vi "linear_backward.vi"(4 "cache":T1, 5 "dZ":dbl[][](array[numeric])) -> (0 "db":dbl[][](array[numeric]), 1 "dW":dbl[][](array[numeric]), 2 "dA_prev":dbl[][](array[numeric]))   [LabVIEW 2020]
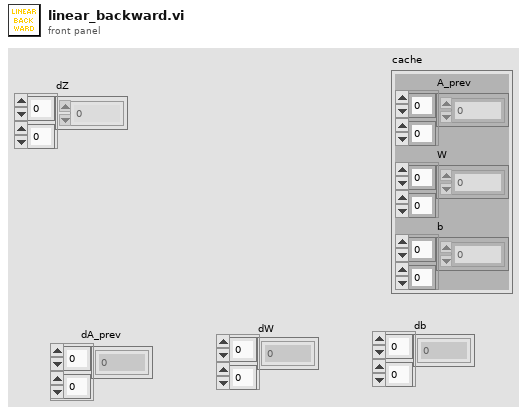
[diagram p1: front panel]
types:
  T1 = cluster{"A_prev":dbl[][], "W":dbl[][], "b":dbl[][]}
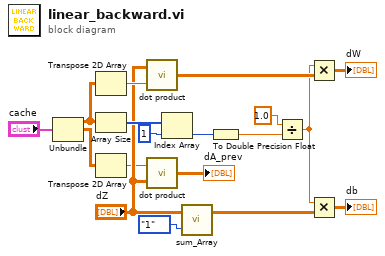
[diagram p0: block diagram]
diagram:
  n1 = Unbundle("cache") -> ("A_prev"=w12:dbl[][], "W"=w6:dbl[][])  [unwired: 1 out]
  n2 = Transpose 2D Array(2D array=w12) -> (transposed array=w11:dbl[][])
  n3 = Array Size(array=w12) -> (size(s)=w17:i32[])
  n4 = Transpose 2D Array(2D array=w6) -> (transposed array=w5:dbl[][])
  n5 = call "dot product.vi"("y"=w11, "x"="dZ") -> ("dot(x,y)"=w10:dbl[][])
  n6 = call "dot product.vi"("y"="dZ", "x"=w5) -> ("dot(x,y)"=→"dA_prev":dbl[][])
  n7 = Index Array(array=w17, index=1) -> (element=w13:i32)
  n8 = call "sum_Array.vi"("axis"=enum16{"None", "0", "1"}."1", "z"="dZ") -> ("sum"=w1:dbl[][])  [unwired: 1 out]
  n9 = To Double Precision Float(number=w13) -> (double precision float=w14:dbl)
  n10 = Divide(x=1.0, y=w14) -> (x/y=w2:dbl)
  n11 = Multiply(x=w2, y=w10) -> (x*y=→"dW":dbl[][])
  n12 = Multiply(x=w2, y=w1) -> (x*y=→"db":dbl[][])
